vi "Overwrite Measurement Role.vi"(0 "Instrument Specifications in":T2, 1 "Measurement Role":T1, 2 "Index":i32, 3 "error in (no error)":errorcluster) -> (7 "Instrument Specifications out":T2, 10 "error out":errorcluster)   [LabVIEW 2026, in "Settings.lvlib"]
uses:
  Settings.lvlib
  Acquisition/Instrument Specifications Configuration.ctl
  Acquisition/Instrument Specifications Cluster Configuration.ctl
  controls/UI/Measurement Role.ctl
  Acquisition/Acquisition.lvlib
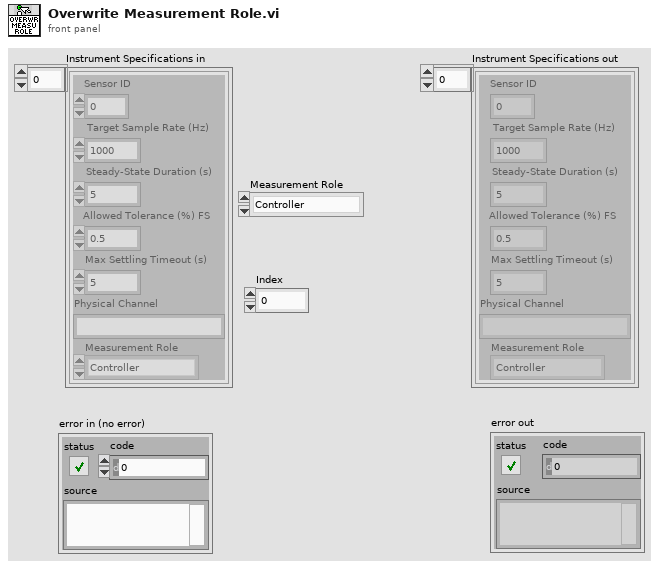
[diagram p1: front panel]
types:
  T1 = typedef "Settings.lvlib/Measurement Role.ctl" = enum16{"Controller", "Reference", "UUT", "Disable", "All"}
  T2 = typedef "Acquisition.lvlib/Instrument Specifications Configuration.ctl" = T3[]
  T3 = typedef "Acquisition.lvlib/Instrument Specifications Cluster Configuration.ctl" = cluster{"Sensor ID":i32, "Target Sample Rate (Hz)":dbl, "Steady-State Duration (s)":i32, "Allowed Tolerance (%) FS":dbl, "Max Settling Timeout (s)":i32, "Physical Channel":string, "Measurement Role":T1}
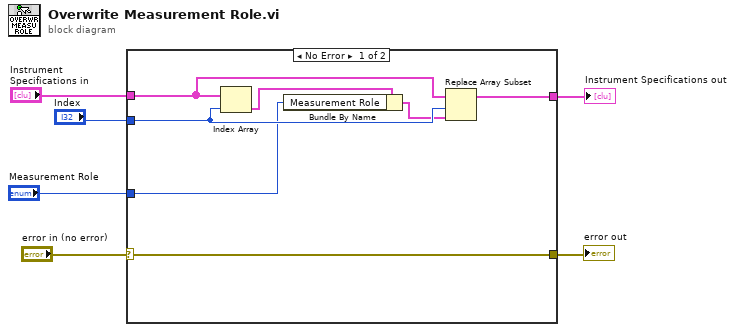
[diagram p0: block diagram]
diagram:
  n1 = case shown="No Error" "error in (no error)" {
    selector: "error in (no error)" -> [w10 w15]
    tunnel: [w13 w14] -> w6
    tunnel: "Index" -> [w12 _]
    tunnel: "Instrument Specifications in" -> [w11 w14]
    tunnel: [w10 w15] -> w2
    tunnel: "Measurement Role" -> [w7 _]
    frame No Error {
      n2 = Index Array(array=w11, index=w12) -> (element=w8:T3)
      n3 = Bundle By Name(cluster=w8, "Measurement Role"=w7) -> (w9:T3)
      n4 = Replace Array Subset(array=w11, new element=w9, index=w12) -> (w13:T2)
    }
    frame Error {
    }
  }
  "Instrument Specifications out" <- w6
  "error out" <- w2
